vi "Actor Core.vi"(8 "error in":errorcluster, 11 "CS++DMMGui.lvclass":refnum<class "CS++DMMGui.lvclass">) -> (0 "error out":errorcluster, 3 "Actor out":refnum<class "Actor.lvclass">)   [LabVIEW 2014, in "CS++DMMGui.lvlib" / "CS++DMMGui.lvclass"]
doc: "(<B>Filename</B>: Actor Framework.lvlib:Actor.lvclass:Actor Core.vi)\n\nReceives messages to the actor, reacts to them, and initiates any error handling that may shut the actor down.\n\nDescendant classes may override this VI to append parallel tasks for the actor to complete while it handles messages. Overrides use the Call Parent Method node."
uses:
  CS++DMMGui.lvclass
  <vilib>/ActorFramework/Actor/Actor.lvclass
  CSPP_Core/Actors/CS++SVMonitor/CS++SVMonitor.lvclass
  CSPP_Core/Classes/CS++ProcessVariables/ProcessVariable/PV.lvclass
  CSPP_Core/Actors/CS++BaseActor/CS++BaseActor.lvclass/CS++BaseActor.ctl
  <vilib>/ActorFramework/Actor/Actor.lvclass/Actor.ctl
  <vilib>/ActorFramework/Message Enqueuer/Message Enqueuer.lvclass/Message Enqueuer.ctl
  CSPP_Core/Actors/CS++DeviceGUIActor/CS++DeviceGUIActor.lvclass/CS++DeviceGUIActor.ctl
  CSPP_Core/Actors/CS++GUIActor/CS++GUIActor.lvclass/CS++GUIActor.ctl
  CS++DMMGui Messages/UpdatePV/UpdatePV.lvclass
  CS++DMMGui.lvclass/CS++DMMGui.ctl
  CSPP_Core/Actors/CS++PVMonitor Messages/Register PVs Msg/Register PVs Msg.lvclass/Register PVs Msg.ctl
  CSPP_Core/Classes/CS++ProcessVariables/ProcessVariable/PV.lvclass/PV.ctl
  CS++DMM Messages/Configure Measurement Msg/Configure Measurement Msg.lvclass/Configure Measurement Msg.ctl
  CS++DMM Messages/Configure AC Bandwidth [AC] Msg/Configure AC Bandwidth [AC] Msg.lvclass/Configure AC Bandwidth [AC] Msg.ctl
  CS++DMM Messages/Configure Frequency Voltage Range [FVR] Msg/Configure Frequency Voltage Range [FVR] Msg.lvclass/Configure Frequency Voltage Range [FVR] Msg.ctl
  CS++DMM Messages/Configure Tranducer Type [TMP] Msg/Configure Tranducer Type [TMP] Msg.lvclass/Configure Tranducer Type [TMP] Msg.ctl
  CS++DMM Messages/Configure Thermocouple [TC] Msg/Configure Thermocouple [TC] Msg.lvclass/Configure Thermocouple [TC] Msg.ctl
  CS++DMM Messages/Configure Fixed Ref Junction [TC] Msg/Configure Fixed Ref Junction [TC] Msg.lvclass/Configure Fixed Ref Junction [TC] Msg.ctl
  CS++DMM Messages/Configure RTD [RTD] Msg/Configure RTD [RTD] Msg.lvclass/Configure RTD [RTD] Msg.ctl
  CS++DMM Messages/Configure Thermistor [THM] Msg/Configure Thermistor [THM] Msg.lvclass/Configure Thermistor [THM] Msg.ctl
  CS++DMM Messages/Configure Trigger Msg/Configure Trigger Msg.lvclass/Configure Trigger Msg.ctl
  CS++DMM Messages/Configure Trigger Slope [TS] Msg/Configure Trigger Slope [TS] Msg.lvclass/Configure Trigger Slope [TS] Msg.ctl
  CS++DMM Messages/Configure Multi-Point [MP] Msg/Configure Multi-Point [MP] Msg.lvclass/Configure Multi-Point [MP] Msg.ctl
  CS++DMM Messages/Configure Meas Complete Dest [MP] Msg/Configure Meas Complete Dest [MP] Msg.lvclass/Configure Meas Complete Dest [MP] Msg.ctl
  CS++DMM Messages/Configure Auto Zero Mode [AZ] Msg/Configure Auto Zero Mode [AZ] Msg.lvclass/Configure Auto Zero Mode [AZ] Msg.ctl
  CS++DMM Messages/Configure Power Line Frequency [PLF] Msg/Configure Power Line Frequency [PLF] Msg.lvclass/Configure Power Line Frequency [PLF] Msg.ctl
  CSPP_Core/Actors/CS++DeviceGUIActor/Read Resource Name.vi
  CSPP_Core/Actors/CS++DeviceGUIActor/Read Driver Revision.vi
  CSPP_Core/Actors/CS++DeviceGUIActor/Read Firmware Revision.vi
  CSPP_Core/Actors/CS++DeviceGUIActor/Read Self-Test Result Code.vi
  CSPP_Core/Actors/CS++DeviceGUIActor/Read Self-Test Result Message.vi
  CSPP_Core/Classes/CS++ProcessVariables/ProcessVariable/Read Data.vi
  <vilib>/ActorFramework/Message Enqueuer/Init from Existing Queue.vi
  <vilib>/ActorFramework/Message Enqueuer/Enqueue.vi
  <vilib>/ActorFramework/Message Priority Queue/Priority Enqueue.vi
  <vilib>/ActorFramework/Message Enqueuer/Message Enqueuer.lvclass
  CSPP_Core/Classes/CS++BaseClasses/Factory/CS++Factory.lvclass
  CSPP_Core/Actors/CS++PVMonitor Messages/Register PVs Msg/Register PVs Msg.lvclass
  <vilib>/ActorFramework/Stop Msg/Stop Msg.lvclass
  CS++DMM Messages/Configure Measurement Msg/Configure Measurement Msg.lvclass
  CS++DMM Messages/Configure AC Bandwidth [AC] Msg/Configure AC Bandwidth [AC] Msg.lvclass
  CS++DMM Messages/Configure Frequency Voltage Range [FVR] Msg/Configure Frequency Voltage Range [FVR] Msg.lvclass
  CS++DMM Messages/Configure Tranducer Type [TMP] Msg/Configure Tranducer Type [TMP] Msg.lvclass
  CS++DMM Messages/Configure Thermocouple [TC] Msg/Configure Thermocouple [TC] Msg.lvclass
  CS++DMM Messages/Configure Fixed Ref Junction [TC] Msg/Configure Fixed Ref Junction [TC] Msg.lvclass
  CS++DMM Messages/Configure RTD [RTD] Msg/Configure RTD [RTD] Msg.lvclass
  CS++DMM Messages/Configure Thermistor [THM] Msg/Configure Thermistor [THM] Msg.lvclass
  CS++DMM Messages/Configure Trigger Msg/Configure Trigger Msg.lvclass
  CS++DMM Messages/Configure Trigger Slope [TS] Msg/Configure Trigger Slope [TS] Msg.lvclass
  CS++DMM Messages/Configure Multi-Point [MP] Msg/Configure Multi-Point [MP] Msg.lvclass
  CS++DMM Messages/Configure Meas Complete Dest [MP] Msg/Configure Meas Complete Dest [MP] Msg.lvclass
  CS++DMM Messages/Configure Auto Zero Mode [AZ] Msg/Configure Auto Zero Mode [AZ] Msg.lvclass
  CS++DMM Messages/Configure Power Line Frequency [PLF] Msg/Configure Power Line Frequency [PLF] Msg.lvclass
  CSPP_Core/Actors/CS++DeviceGUIActor/CS++DeviceGUIActor.lvclass
  CSPP_Core/Actors/CS++BaseActor/CS++BaseActor.lvclass
  CSPP_Core/Actors/CS++GUIActor/CS++GUIActor.lvclass
panel:
  in  "Tab Control":T1(tab)=enum."Configuration"
  out "Associated Actor":string
  out "Driver Revision":string
  out "Firmware Revision":string
  out "Self-Test Result Code":i32
  out "Self-Test Result Message":string
  out "Resource Name":string
  in  "Configuration Tab":T2(tab)
  in  "Config AC Frequency Limits":bool
  in  "AC Max Frequency":dbl=300000.0 caption="ac max frequency (300.0E+3 Hz)" format="%^.2e"
  in  "AC Min Frequency":dbl=20.0 caption="ac min frequency (20.0 Hz)" format="%^.2e"
  in  "Config Measurement":bool
  in  "Range":dbl=-1.0 caption="range (-1.0: Auto)" format="%^.2e"
  in  "Absolute Resolution":dbl=0.001 caption="absolute resolution (0.001)" format="%^.2e"
  out "Actual Range":dbl caption="actual range" format="%^.2e"
  in  "Measurement Function":i32(ring)=1 caption="measurement function (DC Volts)" items=["DC Volts"=1, "AC Volts"=2, "DC Current"=3, "AC Current"=4, "2 Wire Resistance"=5, "4 Wire Resistance"=101, "AC + DC Volts"=106, "AC + DC Current"=107, "Frequency"=104, "Period"=105, "Temperature"=108]
  out "Aperture Time Units":i32 caption="aperture time units"
  out "Aperture Time":dbl caption="aperture time (sec)" format="%^.2e"
  in  "Frequency Volt Range":dbl=10.0 caption="freq volt range (10.0 V RMS)" format="%^.2e"
  in  "Auto Zero Mode":i32(ring) caption="auto zero mode (Off)" items=["On"=1, "Off"=0, "Once"=2]
  in  "Power Line Frequency":dbl[unit]=50.0 caption="power line frequency (60.0 Hz)" format="%^.2e"
  in  "Config RTD":bool
  in  "RTD Alpha":dbl caption="alpha (0.0)" format="%^.2e"
  in  "RTD Resistance":dbl[unit] caption="resistance (0.0 ohms)" format="%^.2e"
  in  "Thermistor Resistance":dbl[unit] caption="resistance (0.0 ohms)" format="%^.2e"
  in  "Transducer Type":i32(ring)=1 caption="transducer type (Thermocouple)" items=["Thermocouple"=1, "Thermistor"=2, "2-Wire RTD"=3, "4-Wire RTD"=4]
  in  "Thermocouple Type":i32(ring)=1 caption="thermocouple type (B)" items=["B"=1, "C"=2, "D"=3, "E"=4, "G"=5, "J"=6, "K"=7, "N"=8, "R"=9, "S"=10, "T"=11, "U"=12, "V"=13]
  in  "Ref Junc Type":i32(ring)=1 caption="ref junc type (Internal)" items=["Internal"=1, "Fixed"=2]
  in  "Fixed Ref Junc":dbl caption="fixed ref junc (0.0 Celsius)" format="%^.2e"
  in  "Config Thermocouple":bool
  in  "Config Trigger":bool
  in  "Trigger Source":i32(ring)=1 caption="trigger source (Immediate)" items=["Immediate"=1, "External"=2, "Software Trigger Function"=3, "PXI TRIG0 or VXI TTL0"=111, "PXI TRIG1 or VXI TTL1"=112, "PXI TRIG2 or VXI TTL2"=113, "PXI TRIG3 or VXI TTL3"=114, "PXI TRIG4 or VXI TTL4"=115, "PXI TRIG5 or VXI TTL5"=116, "PXI TRIG6 or VXI TTL6"=117, "PXI TRIG7 or VXI TTL7"=118, "ECL0"=119, "ECL1"=120, "PXI Star"=131, "RTSI 0"=140, "RTSI 1"=141, "RTSI 2"=142, "RTSI 3"=143, "RTSI 4"=144, "RTSI 5"=145, "RTSI 6"=146]
  in  "Trigger Delay":dbl[unit] caption="trigger delay (0.0 s)" format="%.3f"
  in  "Trigger Slope":i32(ring) caption="trigger slope (0: Positive)" items=["Positive", "Negative"]
  in  "Config MP":bool
  in  "Sample Interval":dbl[unit] caption="sample interval (0.0 s)" format="%.3f"
  in  "Sample Trigger":i32(ring)=1 caption="sample trigger (Immediate)" items=["Immediate"=1, "External"=2, "Software Trigger Function"=3, "Interval"=10, "PXI TRIG0 or VXI TTL0"=111, "PXI TRIG1 or VXI TTL1"=112, "PXI TRIG2 or VXI TTL2"=113, "PXI TRIG3 or VXI TTL3"=114, "PXI TRIG4 or VXI TTL4"=115, "PXI TRIG5 or VXI TTL5"=116, "PXI TRIG6 or VXI TTL6"=117, "PXI TRIG7 or VXI TTL7"=118, "ECL0"=119, "ECL1"=120, "PXI Star"=131, "RTSI 0"=140, "RTSI 1"=141, "RTSI 2"=142, "RTSI 3"=143, "RTSI 4"=144, "RTSI 5"=145, "RTSI 6"=146]
  in  "Trigger Count":i32=1 caption="trigger count (1)"
  in  "Sample Count":i32=1 caption="sample count (1)"
  in  "Complete Trigger Destination":i32(ring)=-1 caption="meas complete dest (None)" items=["None"=-1, "External"=2, "PXI TRIG0 or VXI TTL0"=111, "PXI TRIG1 or VXI TTL1"=112, "PXI TRIG2 or VXI TTL2"=113, "PXI TRIG3 or VXI TTL3"=114, "PXI TRIG4 or VXI TTL4"=115, "PXI TRIG5 or VXI TTL5"=116, "PXI TRIG6 or VXI TTL6"=117, "PXI TRIG7 or VXI TTL7"=118, "ECL0"=119, "ECL1"=120, "PXI Star"=131, "RTSI 0"=140, "RTSI 1"=141, "RTSI 2"=142, "RTSI 3"=143, "RTSI 4"=144, "RTSI 5"=145, "RTSI 6"=146]
  out "Reading Chart":dbl(graph)
  out "IsOverRange":bool
  out "MPReading Graph":dbl[](graph)
  out "IsOverRange":bool
  in  "Stop Button":bool
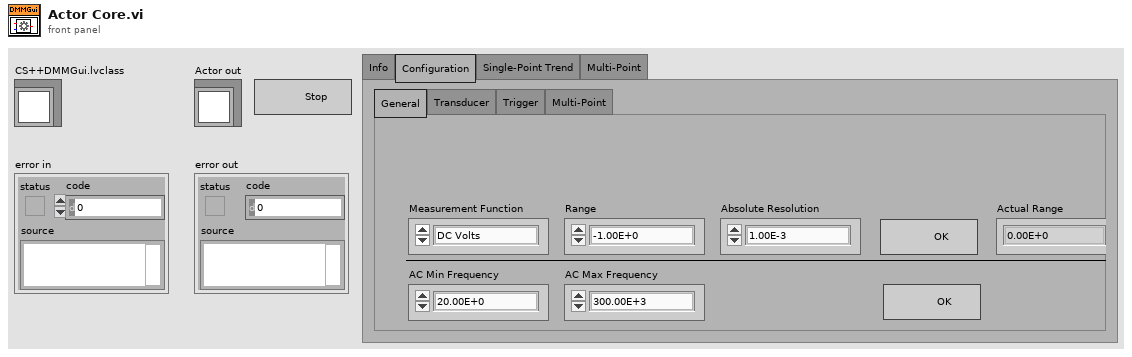
[diagram p1: front panel]
types:
  T1 = enum32{"Info", "Configuration", "Single-Point Trend", "Multi-Point"}
  T2 = enum32{"General", "Transducer", "Trigger", "Multi-Point"}
  T3 = enum32{"Invalid", "Standard", "Closed", "Hidden", "Minimized", "Maximized"}
  T4 = cluster{string, "CS++DMMGui.lvlib:UpdatePV.lvclass":refnum<class "UpdatePV.lvclass">}
  T5 = cluster{"Self Enqueuer":refnum<class "Message Enqueuer.lvclass">, cluster{string, "CS++DMMGui.lvlib:UpdatePV.lvclass":refnum<class "UpdatePV.lvclass">}[]}
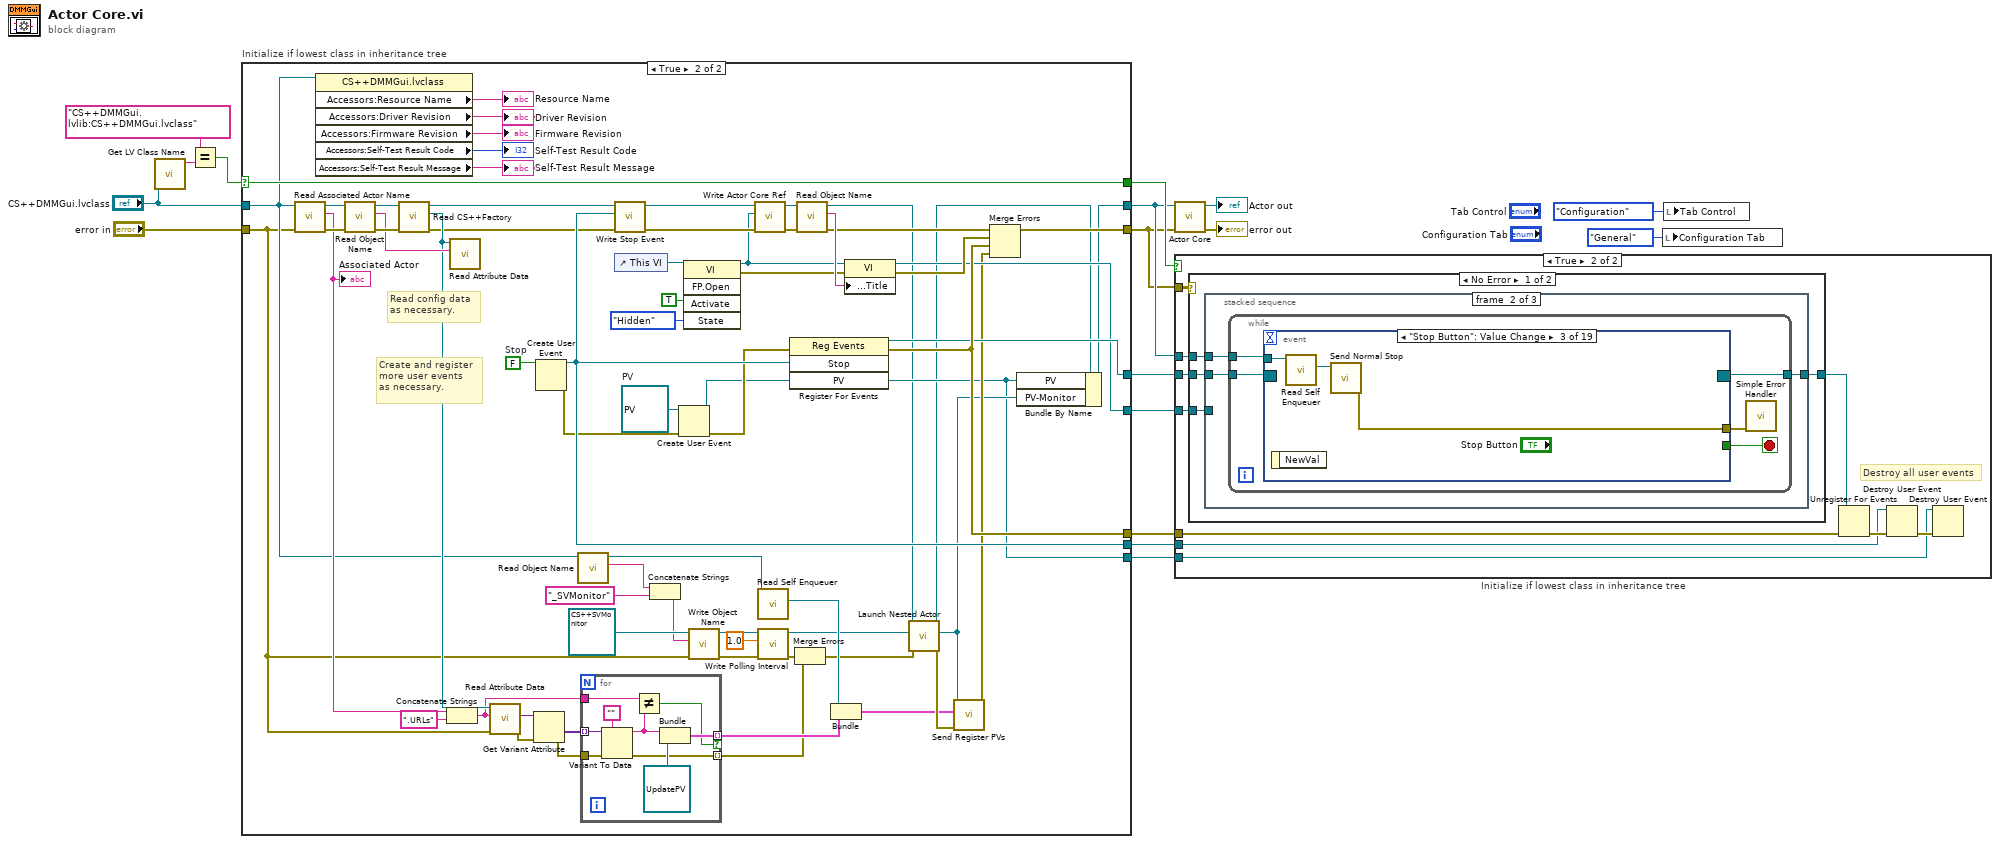
[diagram p0: block diagram]
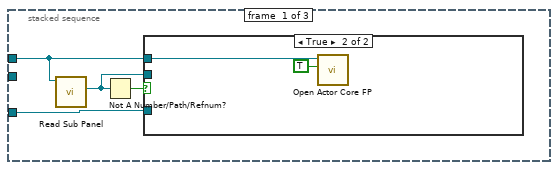
[diagram p4: hidden frame]
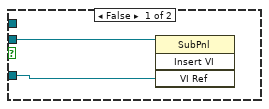
[diagram p5: hidden frame]
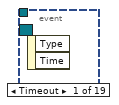
[diagram p6: hidden frame]
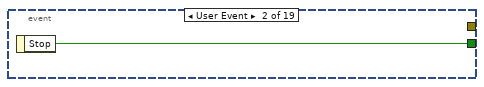
[diagram p7: hidden frame]
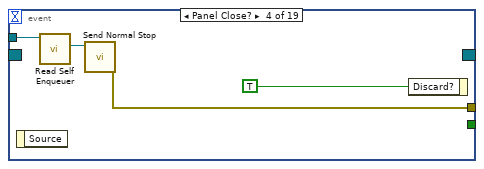
[diagram p8: hidden frame]
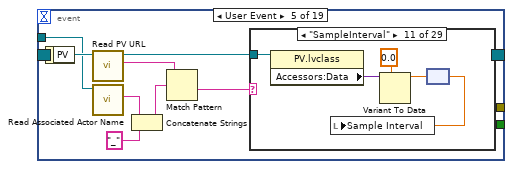
[diagram p9: hidden frame]
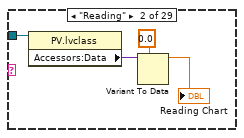
[diagram p11: hidden frame]
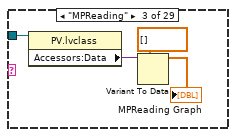
[diagram p12: hidden frame]
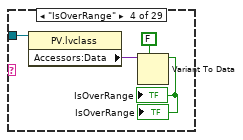
[diagram p13: hidden frame]
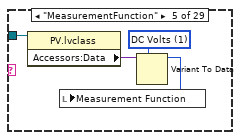
[diagram p14: hidden frame]
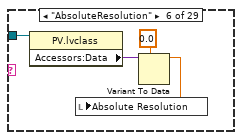
[diagram p15: hidden frame]
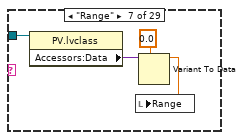
[diagram p16: hidden frame]
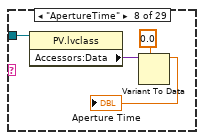
[diagram p17: hidden frame]
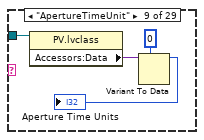
[diagram p18: hidden frame]
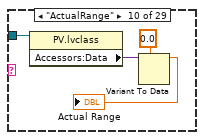
[diagram p19: hidden frame]
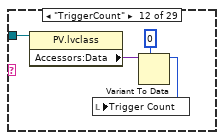
[diagram p20: hidden frame]
diagram:
  n1 = call <vilib>:"Get LV Class Name.vi"("object"="CS++DMMGui.lvclass") -> ("class name"=w15:string)  [unwired: 9 in, 1 out]
  n2 = Equal?(x="CS++DMMGui.lvlib:CS++DMMGui.lvclass" ("class name"), y=w15) -> (x = y?=w9:bool)
  n3 = case "Initialize if lowest class in inheritance tree" shown="True" w9 {
    selector: w9 -> [w18 w62]
    tunnel: [w19 w86] -> w4
    tunnel: "error in" -> [w19 w39]
    tunnel: [w20 w53] -> w5
    tunnel: "CS++DMMGui.lvclass" -> [w20 w41]
    tunnel: [_ w79] -> w13
    tunnel: [_ w78] -> w12
    tunnel: [_ w54] -> w11
    tunnel: [_ w69] -> w10
    tunnel: [w18 w62] -> w8
    tunnel: [_ w34] -> w3
    frame False {
    }
    frame True {
      w38 = refnum<class "PV.lvclass"> refnum  # PV
      w81 = FALSE  # Stop
      # "Create and register \nmore user events\nas necessary."
      # "Read config data\nas necessary."
      n4 = call "Read Associated Actor Name.vi"("error in (no error)"=w39, "CS++GUIActor in"=w41) -> ("error out"=w72:errorcluster, "Associated Actor Name"=w70:string, "CS++GUIActor out"=w73:refnum<class "CS++DMMGui.lvclass">)  [unwired: 7 in]
      "Associated Actor" <- w70
      n5 = property class="CS++DMMGui.lvclass"(reference=w41) -> ("Accessors:Resource Name"=→"Resource Name":string, "Accessors:Driver Revision"=→"Driver Revision":string, "Accessors:Firmware Revision"=→"Firmware Revision":string, "Accessors:Self-Test Result Code"=→"Self-Test Result Code":i32, "Accessors:Self-Test Result Message"=→"Self-Test Result Message":string)  [unwired: 1 in, 2 out]
      n6 = call "Read Object Name.vi"("error in (no error)"=w72, "CS++BaseActor in"=w73) -> ("error out"=w75:errorcluster, "Object Name"=w74:string, "CS++BaseActor out"=w76:refnum<class "CS++DMMGui.lvclass">)  [unwired: 7 in]
      n7 = call "Read CS++Factory.vi"("error in (no error)"=w75, "CS++BaseActor in"=w76) -> ("error out"=w68:errorcluster, "CS++Factory"=w71:refnum<class "CS++Factory.lvclass">, "CS++BaseActor out"=w61:refnum<class "CS++DMMGui.lvclass">)  [unwired: 7 in]
      n8 = Concatenate Strings(w70, ".URLs" ("string")) -> (w24:string)
      n9 = call-dynamic "Read Attribute Data.vi"("Object Name"=w74, "CS++Factory in"=w71) -> ()  [unwired: 7 in, 3 out]
      n10 = call-dynamic "Read Attribute Data.vi"("error in (no error)"=w39, "Object Name"=w24, "CS++Factory in"=w71) -> ("error out"=w28:errorcluster, "Attribute Data"=w27:variant)  [unwired: 6 in, 1 out]
      n11 = Get Variant Attribute(Variant=w27, error in=w28) -> (values=w26:variant[], error out=w25:errorcluster)  [unwired: 2 in, 2 out]
      n12 = Create User Event(user event datatype=w81) -> (user event=w69:refnum<user-event>, error out=w36:errorcluster)  [unwired: 1 in]
      n13 = call "Read Object Name.vi"("CS++BaseActor in"=w41) -> ("Object Name"=w46:string, "CS++BaseActor out"=w45:refnum<class "CS++DMMGui.lvclass">)  [unwired: 8 in, 1 out]
      n14 = for {
        tunnel: [w95] -> w43 mode=indexing if=w91
        tunnel: w26 -> [w94] mode=indexing
        tunnel: w25 -> [w93]
        tunnel: w24 -> [w92]
        tunnel: [w87] -> w31 mode=indexing
        n15 = Variant To Data(error in=w93, type="", Variant=w94) -> (data=w88:string, error out=w87:errorcluster)
        n16 = Not Equal?(x=w92, y=w88) -> (x != y?=w91:bool)
        n17 = Bundle(w88, "CS++DMMGui.lvlib:UpdatePV.lvclass"=refnum<class "UpdatePV.lvclass"> refnum) -> (w95:T4)  [unwired: 1 in]
      }
      n18 = call "Write Stop Event.vi"("error in (no error)"=w68, "Stop"=w69, "CS++GUIActor in"=w61) -> ("error out"=w66:errorcluster, "CS++GUIActor out"=w67:refnum<class "CS++DMMGui.lvclass">)  [unwired: 7 in]
      n19 = control-ref of="This VI"() -> (w85:refnum<vi>)
      n20 = Concatenate Strings(w46, "_SVMonitor" ("Object Name")) -> (w49:string)
      n21 = Create User Event(user event datatype=w38, error in=w36) -> (user event=w34:refnum<user-event>, error out=w35:errorcluster)
      n22 = invoke class="VI" method="FP.Open"(reference=w85, "Activate"=TRUE ("Activate?"), "State"=T3."Hidden") -> (reference out=w55:refnum<vi>, error out=w77:errorcluster)  [unwired: 2 in, 3 out]
      n23 = call "Write Object Name.vi"("error in (no error)"=w39, "Object Name"=w49, "CS++BaseActor in"=refnum<class "CS++SVMonitor.lvclass"> refnum ("CS++SVMonitor.lvlib:CS++SVMonitor.lvclass")) -> ("error out"=w52:errorcluster, "CS++BaseActor out"=w50:refnum<class "CS++SVMonitor.lvclass">)  [unwired: 7 in]
      n24 = call "Write Actor Core Ref.vi"("error in (no error)"=w66, "Actor Core Ref"=w55, "CS++BaseActor in"=w67) -> ("error out"=w65:errorcluster, "CS++BaseActor out"=w64:refnum<class "CS++DMMGui.lvclass">)  [unwired: 7 in]
      n25 = call <vilib>:"Read Self Enqueuer.vi"("Actor"=w45) -> ("Self Enqueuer"=w44:refnum<class "Message Enqueuer.lvclass">)  [unwired: 10 in]
      n26 = call "Write Polling Interval.vi"("error in (no error)"=w52, "Polling Interval"=dbl[unit] 1.0 ("Interval"), "CS++BaseActor in"=w50) -> ("error out"=w32:errorcluster, "CS++BaseActor out"=w23:refnum<class "CS++SVMonitor.lvclass">)  [unwired: 7 in]
      n27 = register-events(error in=w35, w69, w34) -> (reference out=w78:refnum<event-registration>, error out=w79:errorcluster)  [unwired: 1 in]
      n28 = Merge Errors(w32, w31) -> (w30:errorcluster)
      n29 = call "Read Object Name.vi"("error in (no error)"=w65, "CS++BaseActor in"=w64) -> ("error out"=w63:errorcluster, "Object Name"=w82:string, "CS++BaseActor out"=w22:refnum<class "CS++DMMGui.lvclass">)  [unwired: 7 in]
      n30 = Bundle("Self Enqueuer"=w44, w43) -> (w33:T5)  [unwired: 1 in]
      n31 = property class="VI"(reference=w55, error in=w77, "Front Panel.Title"=w82) -> (reference out=w54:refnum<vi>, error out=w80:errorcluster)
      n32 = call <vilib>:"Launch Nested Actor.vi"("error in (no error)"=w30, "Nested Actor"=w23, "Caller Actor in"=w22) -> ("error out"=w42:errorcluster, "Nested Actor's Enqueuer"=w37:refnum<class "Message Enqueuer.lvclass">, "Caller Actor out"=w21:refnum<class "CS++DMMGui.lvclass">)  [unwired: 6 in]
      n33 = call "Send Register PVs.vi"("error in (no error)"=w42, "Register Info"=w33, "Message Enqueuer"=w37) -> ("error out"=w40:errorcluster)  [unwired: 7 in, 1 out]
      n34 = Merge Errors(w63, w80, w79, w40) -> (w86:errorcluster)
      n35 = Bundle By Name(cluster=w21, "PV"=w34, "PV-Monitor"=w37) -> (w53:refnum<class "CS++DMMGui.lvclass">)
    }
  }
  n36 = call-parent "Actor Core.vi"("error in"=w4, "CS++DeviceGUIActor.lvclass"=w5) -> ("error out"=→"error out":errorcluster, "Actor out"=→"Actor out":refnum<class "Actor.lvclass">)  [unwired: 8 in]
  n37 = case "Initialize if lowest class in inheritance tree" shown="True" w8 {
    tunnel: w4 -> [_ w105]
    tunnel: w5 -> [_ w104]
    tunnel: w13 -> [_ w102]
    tunnel: w12 -> [_ w101]
    tunnel: w11 -> [_ w99]
    tunnel: w10 -> [_ w98]
    tunnel: w3 -> [_ w96]
    frame False {
    }
    frame True {
      # "Destroy all user events"
      n38 = case shown="No Error" w105 {
        tunnel: w104 -> [w109 _]
        tunnel: w101 -> [w108 w330]
        tunnel: [w107 w330] -> w100
        tunnel: w99 -> [w106 _]
        frame No Error {
          n39 = stacked-sequence {
            tunnel: w109 -> [w111 w119 w329]
            tunnel: w108 -> [_ w120 _]
            tunnel: [_ w118 _] -> w107
            tunnel: w106 -> [w112 _ _]
            frame #0 {
              n40 = call "Read Sub Panel.vi"("CS++GUIActor in"=w111) -> ("Sub Panel"=w110:refnum<vi>)  [unwired: 8 in, 2 out]
              n41 = Not A Number/Path/Refnum?(number/path/refnum=w110) -> (NaN/Path/Refnum?=w113:bool)
              n42 = case shown="True" w113 {
                tunnel: w111 -> [_ w117]
                tunnel: w110 -> [w115 _]
                tunnel: w112 -> [w114 _]
                frame False {
                  n43 = invoke class="SubPnl" method="Insert VI"(reference=w115, "VI Ref"=w114) -> ()  [unwired: 2 in, 4 out]
                }
                frame True {
                  n44 = call "Open Actor Core FP.vi"("Open FP (F)"=TRUE, "CS++BaseActor in"=w117) -> ()  [unwired: 8 in, 2 out]
                }
              }
            }
            frame #1 {
              n45 = while {
                tunnel: w120 -> [w125]
                tunnel: w119 -> [w124]
                tunnel: [w122] -> w118
                stop <- w123 stop-if-true
                n46 = event shown="[2] \"Stop Button\": Value Change" {
                  selector: w125 -> [_ _ _ _ _ _ _ _ _ _ _ _ _ _ _ _ _ _ _]
                  dyn-events: [_ _ _ _ _ _ _ _ _ _ _ _ _ _ _ _ _ _ _] -> w122
                  timeout: _ -> [_ _ _ _ _ _ _ _ _ _ _ _ _ _ _ _ _ _ _]
                  tunnel: w124 -> [_ _ w129 w131 w139 w262 w266 w272 w276 w281 w285 w291 w295 w302 w306 w314 w318 w322 w327]
                  tunnel: [_ w126 _ _ _ _ _ _ _ _ _ _ _ _ _ _ _ _ _] -> w123
                  tunnel: [_ _ w127 w130 _ w260 w264 w269 w274 w278 w283 w288 w293 w299 w304 w309 w316 w319 w325] -> w121
                  event Timeout {
                    n47 = event-data() -> ()  [unwired: 1 in, 2 out]
                  }
                  event User Event {
                    n48 = event-data() -> ("Stop"=w126:bool)  [unwired: 1 in]
                  }
                  event "Stop Button": Value Change {
                    n49 = event-data() -> ()  [unwired: 1 in, 1 out]
                    n50 = call <vilib>:"Read Self Enqueuer.vi"("Actor"=w129) -> ("Self Enqueuer"=w128:refnum<class "Message Enqueuer.lvclass">)  [unwired: 10 in]
                    n51 = call <vilib>:"Send Normal Stop.vi"("Message Enqueuer"=w128) -> ("error out"=w127:errorcluster)  [unwired: 10 in]
                  }
                  event Panel Close? {
                    n52 = event-data() -> ()  [unwired: 1 in, 1 out]
                    n53 = call <vilib>:"Read Self Enqueuer.vi"("Actor"=w131) -> ("Self Enqueuer"=w132:refnum<class "Message Enqueuer.lvclass">)  [unwired: 10 in]
                    n54 = call <vilib>:"Send Normal Stop.vi"("Message Enqueuer"=w132) -> ("error out"=w130:errorcluster)  [unwired: 10 in]
                    n55 = event-data("Discard?"=TRUE) -> ()  [unwired: 1 in, 1 out]
                  }
                  event User Event {
                    n56 = event-data() -> ("PV"=w141:refnum<class "PV.lvclass">)  [unwired: 1 in]
                    n57 = call "Read PV URL.vi"("PV in"=w141) -> ("PV URL"=w140:string, "PV out"=w135:refnum<class "PV.lvclass">)  [unwired: 8 in, 1 out]
                    n58 = call "Read Associated Actor Name.vi"("CS++GUIActor in"=w139) -> ("Associated Actor Name"=w137:string)  [unwired: 8 in, 2 out]
                    n59 = Concatenate Strings(w137, "_" ("string")) -> (w136:string)
                    n60 = Match Pattern(string=w140, regular expression=w136) -> (after substring=w134:string)  [unwired: 1 in, 3 out]
                    n61 = case shown="\"SampleInterval\"" w134 {
                      tunnel: w135 -> [_ w143 w148 w152 w157 w159 w163 w167 w171 w175 w180 w184 w188 w192 w196 w200 w205 w209 w213 w217 w221 w225 w229 w233 w237 w242 w246 w251 w255]
                      frame Default {
                      }
                      frame "Reading" {
                        n62 = property class="PV.lvclass"(reference=w143) -> ("Accessors:Data"=w145:variant)  [unwired: 1 in, 2 out]
                        n63 = Variant To Data(type=0.0, Variant=w145) -> (data=→"Reading Chart":dbl)  [unwired: 1 in, 1 out]
                      }
                      frame "MPReading" {
                        n64 = property class="PV.lvclass"(reference=w148) -> ("Accessors:Data"=w149:variant)  [unwired: 1 in, 2 out]
                        n65 = Variant To Data(type=dbl[] [], Variant=w149) -> (data=→"MPReading Graph":dbl[])  [unwired: 1 in, 1 out]
                      }
                      frame "IsOverRange" {
                        n66 = property class="PV.lvclass"(reference=w152) -> ("Accessors:Data"=w153:variant)  [unwired: 1 in, 2 out]
                        n67 = Variant To Data(type=FALSE, Variant=w153) -> (data=→"IsOverRange" →"IsOverRange":bool)  [unwired: 1 in, 1 out]
                      }
                      frame "MeasurementFunction" {
                        w154 = 1 items=["DC Volts"=1, "AC Volts"=2, "DC Current"=3, "AC Current"=4, "2 Wire Resistance"=5, "4 Wire Resistance"=101, "AC + DC Volts"=106, "AC + DC Current"=107, "Frequency"=104, "Period"=105, "Temperature"=108] ("measurement function (DC Volts)")
                        n68 = property class="PV.lvclass"(reference=w157) -> ("Accessors:Data"=w156:variant)  [unwired: 1 in, 2 out]
                        n69 = Variant To Data(type=w154, Variant=w156) -> (data=w155:i32)  [unwired: 1 in, 1 out]
                        n70 = local write "Measurement Function"(w155) -> ()
                      }
                      frame "AbsoluteResolution" {
                        n71 = property class="PV.lvclass"(reference=w159) -> ("Accessors:Data"=w160:variant)  [unwired: 1 in, 2 out]
                        n72 = Variant To Data(type=0.0, Variant=w160) -> (data=w158:dbl)  [unwired: 1 in, 1 out]
                        n73 = local write "Absolute Resolution"(w158) -> ()
                      }
                      frame "Range" {
                        n74 = property class="PV.lvclass"(reference=w163) -> ("Accessors:Data"=w164:variant)  [unwired: 1 in, 2 out]
                        n75 = Variant To Data(type=0.0, Variant=w164) -> (data=w162:dbl)  [unwired: 1 in, 1 out]
                        n76 = local write "Range"(w162) -> ()
                      }
                      frame "ApertureTime" {
                        n77 = property class="PV.lvclass"(reference=w167) -> ("Accessors:Data"=w168:variant)  [unwired: 1 in, 2 out]
                        n78 = Variant To Data(type=0.0, Variant=w168) -> (data=→"Aperture Time":dbl)  [unwired: 1 in, 1 out]
                      }
                      frame "ApertureTimeUnit" {
                        n79 = property class="PV.lvclass"(reference=w171) -> ("Accessors:Data"=w172:variant)  [unwired: 1 in, 2 out]
                        n80 = Variant To Data(type=0, Variant=w172) -> (data=→"Aperture Time Units":i32)  [unwired: 1 in, 1 out]
                      }
                      frame "ActualRange" {
                        n81 = property class="PV.lvclass"(reference=w175) -> ("Accessors:Data"=w176:variant)  [unwired: 1 in, 2 out]
                        n82 = Variant To Data(type=0.0, Variant=w176) -> (data=→"Actual Range":dbl)  [unwired: 1 in, 1 out]
                      }
                      frame "SampleInterval" {
                        n83 = property class="PV.lvclass"(reference=w180) -> ("Accessors:Data"=w181:variant)  [unwired: 1 in, 2 out]
                        n84 = Variant To Data(type=0.0, Variant=w181) -> (data=w179:dbl)  [unwired: 1 in, 1 out]
                        n85 = node(w179) -> (w178:dbl[unit])
                        n86 = local write "Sample Interval"(w178) -> ()
                      }
                      frame "TriggerCount" {
                        n87 = property class="PV.lvclass"(reference=w184) -> ("Accessors:Data"=w185:variant)  [unwired: 1 in, 2 out]
                        n88 = Variant To Data(type=0, Variant=w185) -> (data=w183:i32)  [unwired: 1 in, 1 out]
                        n89 = local write "Trigger Count"(w183) -> ()
                      }
                      frame "SampleCount" {
                        n90 = property class="PV.lvclass"(reference=w188) -> ("Accessors:Data"=w189:variant)  [unwired: 1 in, 2 out]
                        n91 = Variant To Data(type=0, Variant=w189) -> (data=w187:i32)  [unwired: 1 in, 1 out]
                        n92 = local write "Sample Count"(w187) -> ()
                      }
                      frame "SampleTrigger" {
                        n93 = property class="PV.lvclass"(reference=w192) -> ("Accessors:Data"=w193:variant)  [unwired: 1 in, 2 out]
                        n94 = Variant To Data(type=0, Variant=w193) -> (data=w191:i32)  [unwired: 1 in, 1 out]
                        n95 = local write "Sample Trigger"(w191) -> ()
                      }
                      frame "MeasCompleteDestination" {
                        n96 = property class="PV.lvclass"(reference=w196) -> ("Accessors:Data"=w197:variant)  [unwired: 1 in, 2 out]
                        n97 = Variant To Data(type=0, Variant=w197) -> (data=w195:i32)  [unwired: 1 in, 1 out]
                        n98 = local write "Complete Trigger Destination"(w195) -> ()
                      }
                      frame "AutoZeroMode" {
                        n99 = property class="PV.lvclass"(reference=w200) -> ("Accessors:Data"=w201:variant)  [unwired: 1 in, 2 out]
                        n100 = Variant To Data(type=0, Variant=w201) -> (data=w199:i32)  [unwired: 1 in, 1 out]
                        n101 = local write "Auto Zero Mode"(w199) -> ()
                      }
                      frame "PowerLineFrequency" {
                        n102 = property class="PV.lvclass"(reference=w205) -> ("Accessors:Data"=w206:variant)  [unwired: 1 in, 2 out]
                        n103 = Variant To Data(type=0.0, Variant=w206) -> (data=w204:dbl)  [unwired: 1 in, 1 out]
                        n104 = node(w204) -> (w203:dbl[unit])
                        n105 = local write "Power Line Frequency"(w203) -> ()
                      }
                      frame "FrequencyVoltageRange" {
                        n106 = property class="PV.lvclass"(reference=w209) -> ("Accessors:Data"=w210:variant)  [unwired: 1 in, 2 out]
                        n107 = Variant To Data(type=0.0, Variant=w210) -> (data=w208:dbl)  [unwired: 1 in, 1 out]
                        n108 = local write "Frequency Volt Range"(w208) -> ()
                      }
                      frame "ACMinFrequency" {
                        n109 = property class="PV.lvclass"(reference=w213) -> ("Accessors:Data"=w214:variant)  [unwired: 1 in, 2 out]
                        n110 = Variant To Data(type=0.0, Variant=w214) -> (data=w212:dbl)  [unwired: 1 in, 1 out]
                        n111 = local write "AC Min Frequency"(w212) -> ()
                      }
                      frame "ACMaxFrequency" {
                        n112 = property class="PV.lvclass"(reference=w217) -> ("Accessors:Data"=w218:variant)  [unwired: 1 in, 2 out]
                        n113 = Variant To Data(type=0.0, Variant=w218) -> (data=w216:dbl)  [unwired: 1 in, 1 out]
                        n114 = local write "AC Max Frequency"(w216) -> ()
                      }
                      frame "TransducerType" {
                        n115 = property class="PV.lvclass"(reference=w221) -> ("Accessors:Data"=w222:variant)  [unwired: 1 in, 2 out]
                        n116 = Variant To Data(type=0, Variant=w222) -> (data=w220:i32)  [unwired: 1 in, 1 out]
                        n117 = local write "Transducer Type"(w220) -> ()
                      }
                      frame "ThermocoupleType" {
                        n118 = property class="PV.lvclass"(reference=w225) -> ("Accessors:Data"=w226:variant)  [unwired: 1 in, 2 out]
                        n119 = Variant To Data(type=0, Variant=w226) -> (data=w224:i32)  [unwired: 1 in, 1 out]
                        n120 = local write "Thermocouple Type"(w224) -> ()
                      }
                      frame "ReferenceJunctionType" {
                        n121 = property class="PV.lvclass"(reference=w229) -> ("Accessors:Data"=w230:variant)  [unwired: 1 in, 2 out]
                        n122 = Variant To Data(type=0, Variant=w230) -> (data=w228:i32)  [unwired: 1 in, 1 out]
                        n123 = local write "Ref Junc Type"(w228) -> ()
                      }
                      frame "FixedReferenceJunction" {
                        n124 = property class="PV.lvclass"(reference=w233) -> ("Accessors:Data"=w234:variant)  [unwired: 1 in, 2 out]
                        n125 = Variant To Data(type=0.0, Variant=w234) -> (data=w232:dbl)  [unwired: 1 in, 1 out]
                        n126 = local write "Fixed Ref Junc"(w232) -> ()
                      }
                      frame "Alpha" {
                        n127 = property class="PV.lvclass"(reference=w237) -> ("Accessors:Data"=w238:variant)  [unwired: 1 in, 2 out]
                        n128 = Variant To Data(type=0.0, Variant=w238) -> (data=w236:dbl)  [unwired: 1 in, 1 out]
                        n129 = local write "RTD Alpha"(w236) -> ()
                      }
                      frame "Resistance" {
                        n130 = property class="PV.lvclass"(reference=w242) -> ("Accessors:Data"=w243:variant)  [unwired: 1 in, 2 out]
                        n131 = Variant To Data(type=0.0, Variant=w243) -> (data=w241:dbl)  [unwired: 1 in, 1 out]
                        n132 = node(w241) -> (w240:dbl[unit])
                        n133 = local write "Thermistor Resistance"(w240) -> ()
                        n134 = local write "RTD Resistance"(w240) -> ()
                      }
                      frame "TriggerSource" {
                        n135 = property class="PV.lvclass"(reference=w246) -> ("Accessors:Data"=w247:variant)  [unwired: 1 in, 2 out]
                        n136 = Variant To Data(type=0, Variant=w247) -> (data=w245:i32)  [unwired: 1 in, 1 out]
                        n137 = local write "Trigger Source"(w245) -> ()
                      }
                      frame "TriggerDelay" {
                        n138 = property class="PV.lvclass"(reference=w251) -> ("Accessors:Data"=w252:variant)  [unwired: 1 in, 2 out]
                        n139 = Variant To Data(type=0.0, Variant=w252) -> (data=w250:dbl)  [unwired: 1 in, 1 out]
                        n140 = node(w250) -> (w249:dbl[unit])
                        n141 = local write "Trigger Delay"(w249) -> ()
                      }
                      frame "TriggerSlope" {
                        n142 = property class="PV.lvclass"(reference=w255) -> ("Accessors:Data"=w256:variant)  [unwired: 1 in, 2 out]
                        n143 = Variant To Data(type=0, Variant=w256) -> (data=w254:i32)  [unwired: 1 in, 1 out]
                        n144 = local write "Trigger Slope"(w254) -> ()
                      }
                    }
                  }
                  event "Config Measurement": Value Change {
                    n145 = event-data() -> ()  [unwired: 1 in, 2 out]
                    n146 = call "Read Associated Actor Enqueuer.vi"("CS++GUIActor in"=w262) -> ("Associated Actor Enqueuer"=w261:refnum<class "Message Enqueuer.lvclass">)  [unwired: 8 in, 2 out]
                    n147 = call "Send Configure Measurement.vi"("absolute resolution (0.001)"="Absolute Resolution", "range (-1.0: Auto)"="Range", "measurement function (DC Volts)"="Measurement Function", "Message Enqueuer"=w261) -> ("error out"=w260:errorcluster)  [unwired: 6 in, 1 out]
                  }
                  event "Config AC Frequency Limits": Value Change {
                    n148 = event-data() -> ()  [unwired: 1 in, 2 out]
                    n149 = call "Read Associated Actor Enqueuer.vi"("CS++GUIActor in"=w266) -> ("Associated Actor Enqueuer"=w265:refnum<class "Message Enqueuer.lvclass">)  [unwired: 8 in, 2 out]
                    n150 = call "Send Configure AC Bandwidth [AC].vi"("ac max frequency (300.0E+3 Hz)"="AC Max Frequency", "ac min frequency (20.0 Hz)"="AC Min Frequency", "Message Enqueuer"=w265) -> ("error out"=w264:errorcluster)  [unwired: 7 in, 1 out]
                  }
                  event "Frequency Volt Range": Value Change {
                    n151 = event-data() -> ()  [unwired: 1 in, 1 out]
                    n152 = call "Read Associated Actor Enqueuer.vi"("CS++GUIActor in"=w272) -> ("Associated Actor Enqueuer"=w270:refnum<class "Message Enqueuer.lvclass">)  [unwired: 8 in, 2 out]
                    n153 = call "Send Configure Frequency Voltage Range [FVR].vi"("freq volt range (10.0 V RMS)"="Frequency Volt Range", "Message Enqueuer"=w270) -> ("error out"=w269:errorcluster)  [unwired: 8 in, 1 out]
                  }
                  event "Transducer Type": Value Change {
                    n154 = event-data() -> ()  [unwired: 1 in, 1 out]
                    n155 = call "Read Associated Actor Enqueuer.vi"("CS++GUIActor in"=w276) -> ("Associated Actor Enqueuer"=w273:refnum<class "Message Enqueuer.lvclass">)  [unwired: 8 in, 2 out]
                    n156 = call "Send Configure Tranducer Type [TMP].vi"("transducer type (Thermocouple)"="Transducer Type", "Message Enqueuer"=w273) -> ("error out"=w274:errorcluster)  [unwired: 8 in, 1 out]
                  }
                  event "Config Thermocouple": Value Change {
                    n157 = event-data() -> ()  [unwired: 1 in, 2 out]
                    n158 = call "Read Associated Actor Enqueuer.vi"("CS++GUIActor in"=w281) -> ("Associated Actor Enqueuer"=w277:refnum<class "Message Enqueuer.lvclass">)  [unwired: 8 in, 2 out]
                    n159 = call "Send Configure Thermocouple [TC].vi"("ref junc type (Internal)"="Ref Junc Type", "thermocouple type (B)"="Thermocouple Type", "Message Enqueuer"=w277) -> ("error out"=w278:errorcluster)  [unwired: 7 in, 1 out]
                  }
                  event "Fixed Ref Junc": Value Change {
                    n160 = event-data() -> ()  [unwired: 1 in, 1 out]
                    n161 = call "Read Associated Actor Enqueuer.vi"("CS++GUIActor in"=w285) -> ("Associated Actor Enqueuer"=w282:refnum<class "Message Enqueuer.lvclass">)  [unwired: 8 in, 2 out]
                    n162 = call "Send Configure Fixed Ref Junction [TC].vi"("fixed ref junc (0.0 Celsius)"="Fixed Ref Junc", "Message Enqueuer"=w282) -> ("error out"=w283:errorcluster)  [unwired: 8 in, 1 out]
                  }
                  event "Config RTD": Value Change {
                    n163 = event-data() -> ()  [unwired: 1 in, 2 out]
                    n164 = call "Read Associated Actor Enqueuer.vi"("CS++GUIActor in"=w291) -> ("Associated Actor Enqueuer"=w287:refnum<class "Message Enqueuer.lvclass">)  [unwired: 8 in, 2 out]
                    n165 = node("RTD Resistance") -> (w286:dbl)
                    n166 = call "Send Configure RTD [RTD].vi"("resistance (0.0 ohms)"=w286, "alpha (0.0)"="RTD Alpha", "Message Enqueuer"=w287) -> ("error out"=w288:errorcluster)  [unwired: 7 in, 1 out]
                  }
                  event "Thermistor Resistance": Value Change {
                    n167 = event-data() -> ()  [unwired: 1 in, 1 out]
                    n168 = call "Read Associated Actor Enqueuer.vi"("CS++GUIActor in"=w295) -> ("Associated Actor Enqueuer"=w294:refnum<class "Message Enqueuer.lvclass">)  [unwired: 8 in, 2 out]
                    n169 = node("Thermistor Resistance") -> (w292:dbl)
                    n170 = call "Send Configure Thermistor [THM].vi"("resistance (0.0 ohms)"=w292, "Message Enqueuer"=w294) -> ("error out"=w293:errorcluster)  [unwired: 8 in, 1 out]
                  }
                  event "Config Trigger": Value Change {
                    n171 = event-data() -> ()  [unwired: 1 in, 2 out]
                    n172 = call "Read Associated Actor Enqueuer.vi"("CS++GUIActor in"=w302) -> ("Associated Actor Enqueuer"=w298:refnum<class "Message Enqueuer.lvclass">)  [unwired: 8 in, 2 out]
                    n173 = node("Trigger Delay") -> (w297:dbl)
                    n174 = call "Send Configure Trigger.vi"("trigger delay (0.0 s)"=w297, "trigger source (Immediate)"="Trigger Source", "Message Enqueuer"=w298) -> ("error out"=w299:errorcluster)  [unwired: 7 in, 1 out]
                  }
                  event "Trigger Slope": Value Change {
                    n175 = event-data() -> ()  [unwired: 1 in, 1 out]
                    n176 = call "Read Associated Actor Enqueuer.vi"("CS++GUIActor in"=w306) -> ("Associated Actor Enqueuer"=w303:refnum<class "Message Enqueuer.lvclass">)  [unwired: 8 in, 2 out]
                    n177 = call "Send Configure Trigger Slope [TS].vi"("trigger slope (0: Positive)"="Trigger Slope", "Message Enqueuer"=w303) -> ("error out"=w304:errorcluster)  [unwired: 8 in, 1 out]
                  }
                  event "Config MP": Value Change {
                    n178 = event-data() -> ()  [unwired: 1 in, 2 out]
                    n179 = call "Read Associated Actor Enqueuer.vi"("CS++GUIActor in"=w314) -> ("Associated Actor Enqueuer"=w308:refnum<class "Message Enqueuer.lvclass">)  [unwired: 8 in, 2 out]
                    n180 = node("Sample Interval") -> (w307:dbl)
                    n181 = call "Send Configure Multi-Point [MP].vi"("sample count (1)"="Sample Count", "trigger count (1)"="Trigger Count", "sample trigger (Immediate)"="Sample Trigger", "sample interval (0.0 s)"=w307, "Message Enqueuer"=w308) -> ("error out"=w309:errorcluster)  [unwired: 5 in, 1 out]
                  }
                  event "Complete Trigger Destination": Value Change {
                    n182 = event-data() -> ()  [unwired: 1 in, 1 out]
                    n183 = call "Read Associated Actor Enqueuer.vi"("CS++GUIActor in"=w318) -> ("Associated Actor Enqueuer"=w315:refnum<class "Message Enqueuer.lvclass">)  [unwired: 8 in, 2 out]
                    n184 = call "Send Configure Meas Complete Dest [MP].vi"("meas complete dest (None)"="Complete Trigger Destination", "Message Enqueuer"=w315) -> ("error out"=w316:errorcluster)  [unwired: 8 in, 1 out]
                  }
                  event "Auto Zero Mode": Value Change {
                    n185 = event-data() -> ()  [unwired: 1 in, 1 out]
                    n186 = call "Read Associated Actor Enqueuer.vi"("CS++GUIActor in"=w322) -> ("Associated Actor Enqueuer"=w320:refnum<class "Message Enqueuer.lvclass">)  [unwired: 8 in, 2 out]
                    n187 = call "Send Configure Auto Zero Mode [AZ].vi"("auto zero mode (Off)"="Auto Zero Mode", "Message Enqueuer"=w320) -> ("error out"=w319:errorcluster)  [unwired: 8 in, 1 out]
                  }
                  event "Power Line Frequency": Value Change {
                    n188 = event-data() -> ()  [unwired: 1 in, 1 out]
                    n189 = call "Read Associated Actor Enqueuer.vi"("CS++GUIActor in"=w327) -> ("Associated Actor Enqueuer"=w324:refnum<class "Message Enqueuer.lvclass">)  [unwired: 8 in, 2 out]
                    n190 = node("Power Line Frequency") -> (w323:dbl)
                    n191 = call "Send Configure Power Line Frequency [PLF].vi"("power line frequency (60.0 Hz)"=w323, "Message Enqueuer"=w324) -> ("error out"=w325:errorcluster)  [unwired: 8 in, 1 out]
                  }
                }
                n192 = call <vilib>:"Simple Error Handler.vi"("error in (no error)"=w121) -> ()  [unwired: 4 in, 5 out]
              }
            }
            frame #2 {
              n193 = call "Open Actor Core FP.vi"("Open FP (F)"=FALSE, "CS++BaseActor in"=w329) -> ()  [unwired: 8 in, 2 out]
            }
          }
        }
        frame Error {
        }
      }
      n194 = Unregister For Events(event registration refnum=w100, error in=w102) -> (error out=w103:errorcluster)
      n195 = Destroy User Event(user event=w98, error in=w103) -> (error out=w97:errorcluster)
      n196 = Destroy User Event(user event=w96, error in=w97) -> ()  [unwired: 1 out]
    }
  }
  n197 = local write "Configuration Tab"(T2."General" ("Configuration Tab")) -> ()
  n198 = local write "Tab Control"(T1."Configuration" ("Tab Control")) -> ()
